vi "satellite simulator control.vi"() -> ()   [LabVIEW 2012]
uses:
  <vilib>/Utility/error.llb/DialogType.ctl
  <vilib>/DAQmx/create/channels.llb/DAQmx Create Channel (DO-Digital Output).vi
  <vilib>/vision/NI_Vision_Development_Module.lvlib
panel:
  in  "Pixel-Distance Ratio (pix/cm)":dbl=8.26
  in  "Remote Logger Status":bool
  in  "Downlink Object Data?":bool
  in  "Remote Port":u16=61557
  in  "Local Port":u16=61556
  in  "Remote Host":string="localhost"
  in  "broadcast":bool
  in  "Maintain Attitude":bool
  out "alpha":dbl
  out "Objects":T1(array[cluster]) {"Aspect Ratio" format="%.2f"; "Orientation" format="%.2f"; "Area" format="%.2f"; "Object Center"."Y" format="%.2f"; "Object Center"."X" format="%.2f"}
  in  "Y Center Correction":dbl
  in  "X Center Correction":dbl
  out "Offset Degree":dbl
  in  "Y Desired":dbl
  in  "X Desired":dbl
  out "Vx (cm/s)":dbl
  out "Vy (cm/s)":dbl
  in  "OK Button":bool
  out "Filtered Ohmega":dbl
  in  "Air Floating Status":bool
  in  "Control Freq":u32=20
  in  "Alpha Desired":dbl
  in  "STOP":bool caption="stop (F)"
  out "Image Out":T2(plugin-control)
  out "alpha (deg)":dbl
  out "dx (cm)":dbl
  out "dy (cm)":dbl
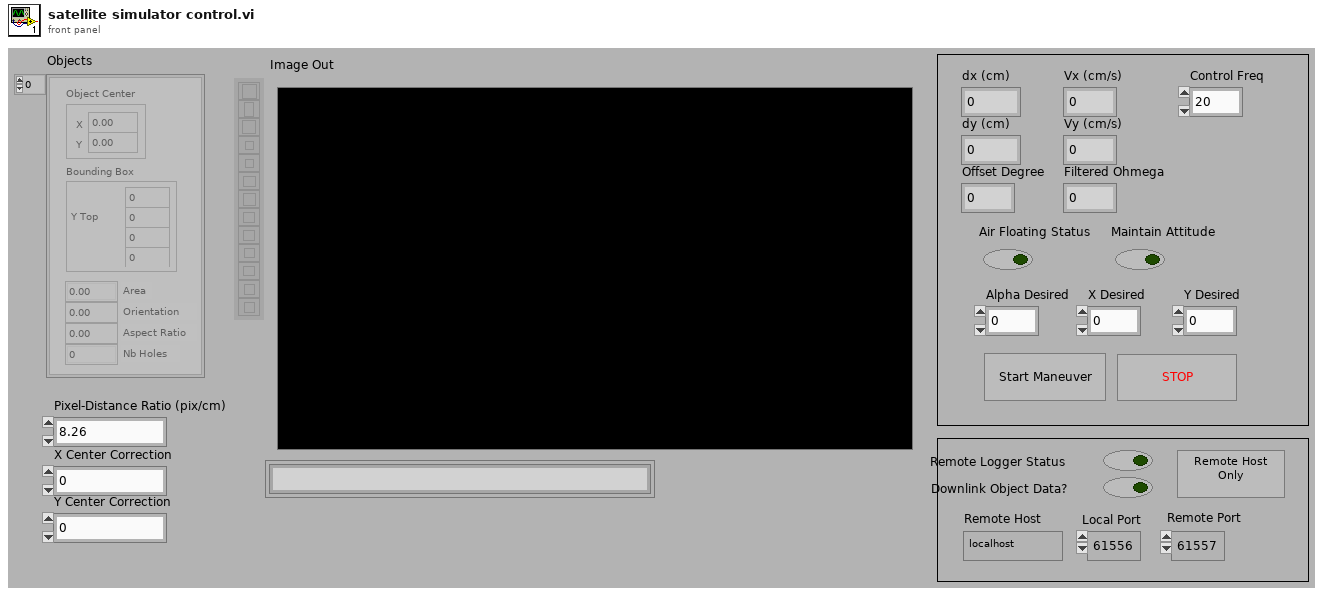
[diagram p1: front panel]
types:
  T1 = cluster{"Object Center":cluster{"X":sgl, "Y":sgl}, "Bounding Box":cluster{"X Left":i32, "Y Top":i32, "X Right":i32, "Y Bottom":i32}, "Area":sgl, "Orientation":sgl, "Aspect Ratio":sgl, "Nb Holes":i32}[]
  T2 = typedef "IMAQ Image.ctl" = refnum<image>
  T3 = typedef "DialogType.ctl" = u16
  T4 = cluster{"dx (cm)":dbl, "dy (cm)":dbl, "Offset Degree":dbl}
  T5 = cluster{"Objects":u16, "Threshold":i32, "Reject Border":bool, "Fill Holes":bool, "Min Object Size":bool, "Min Size":i32, "Max Object Size":bool, "Max Size":i32, "Show Search Area":bool, "Show Center":bool, "Show Bounding Box":bool}
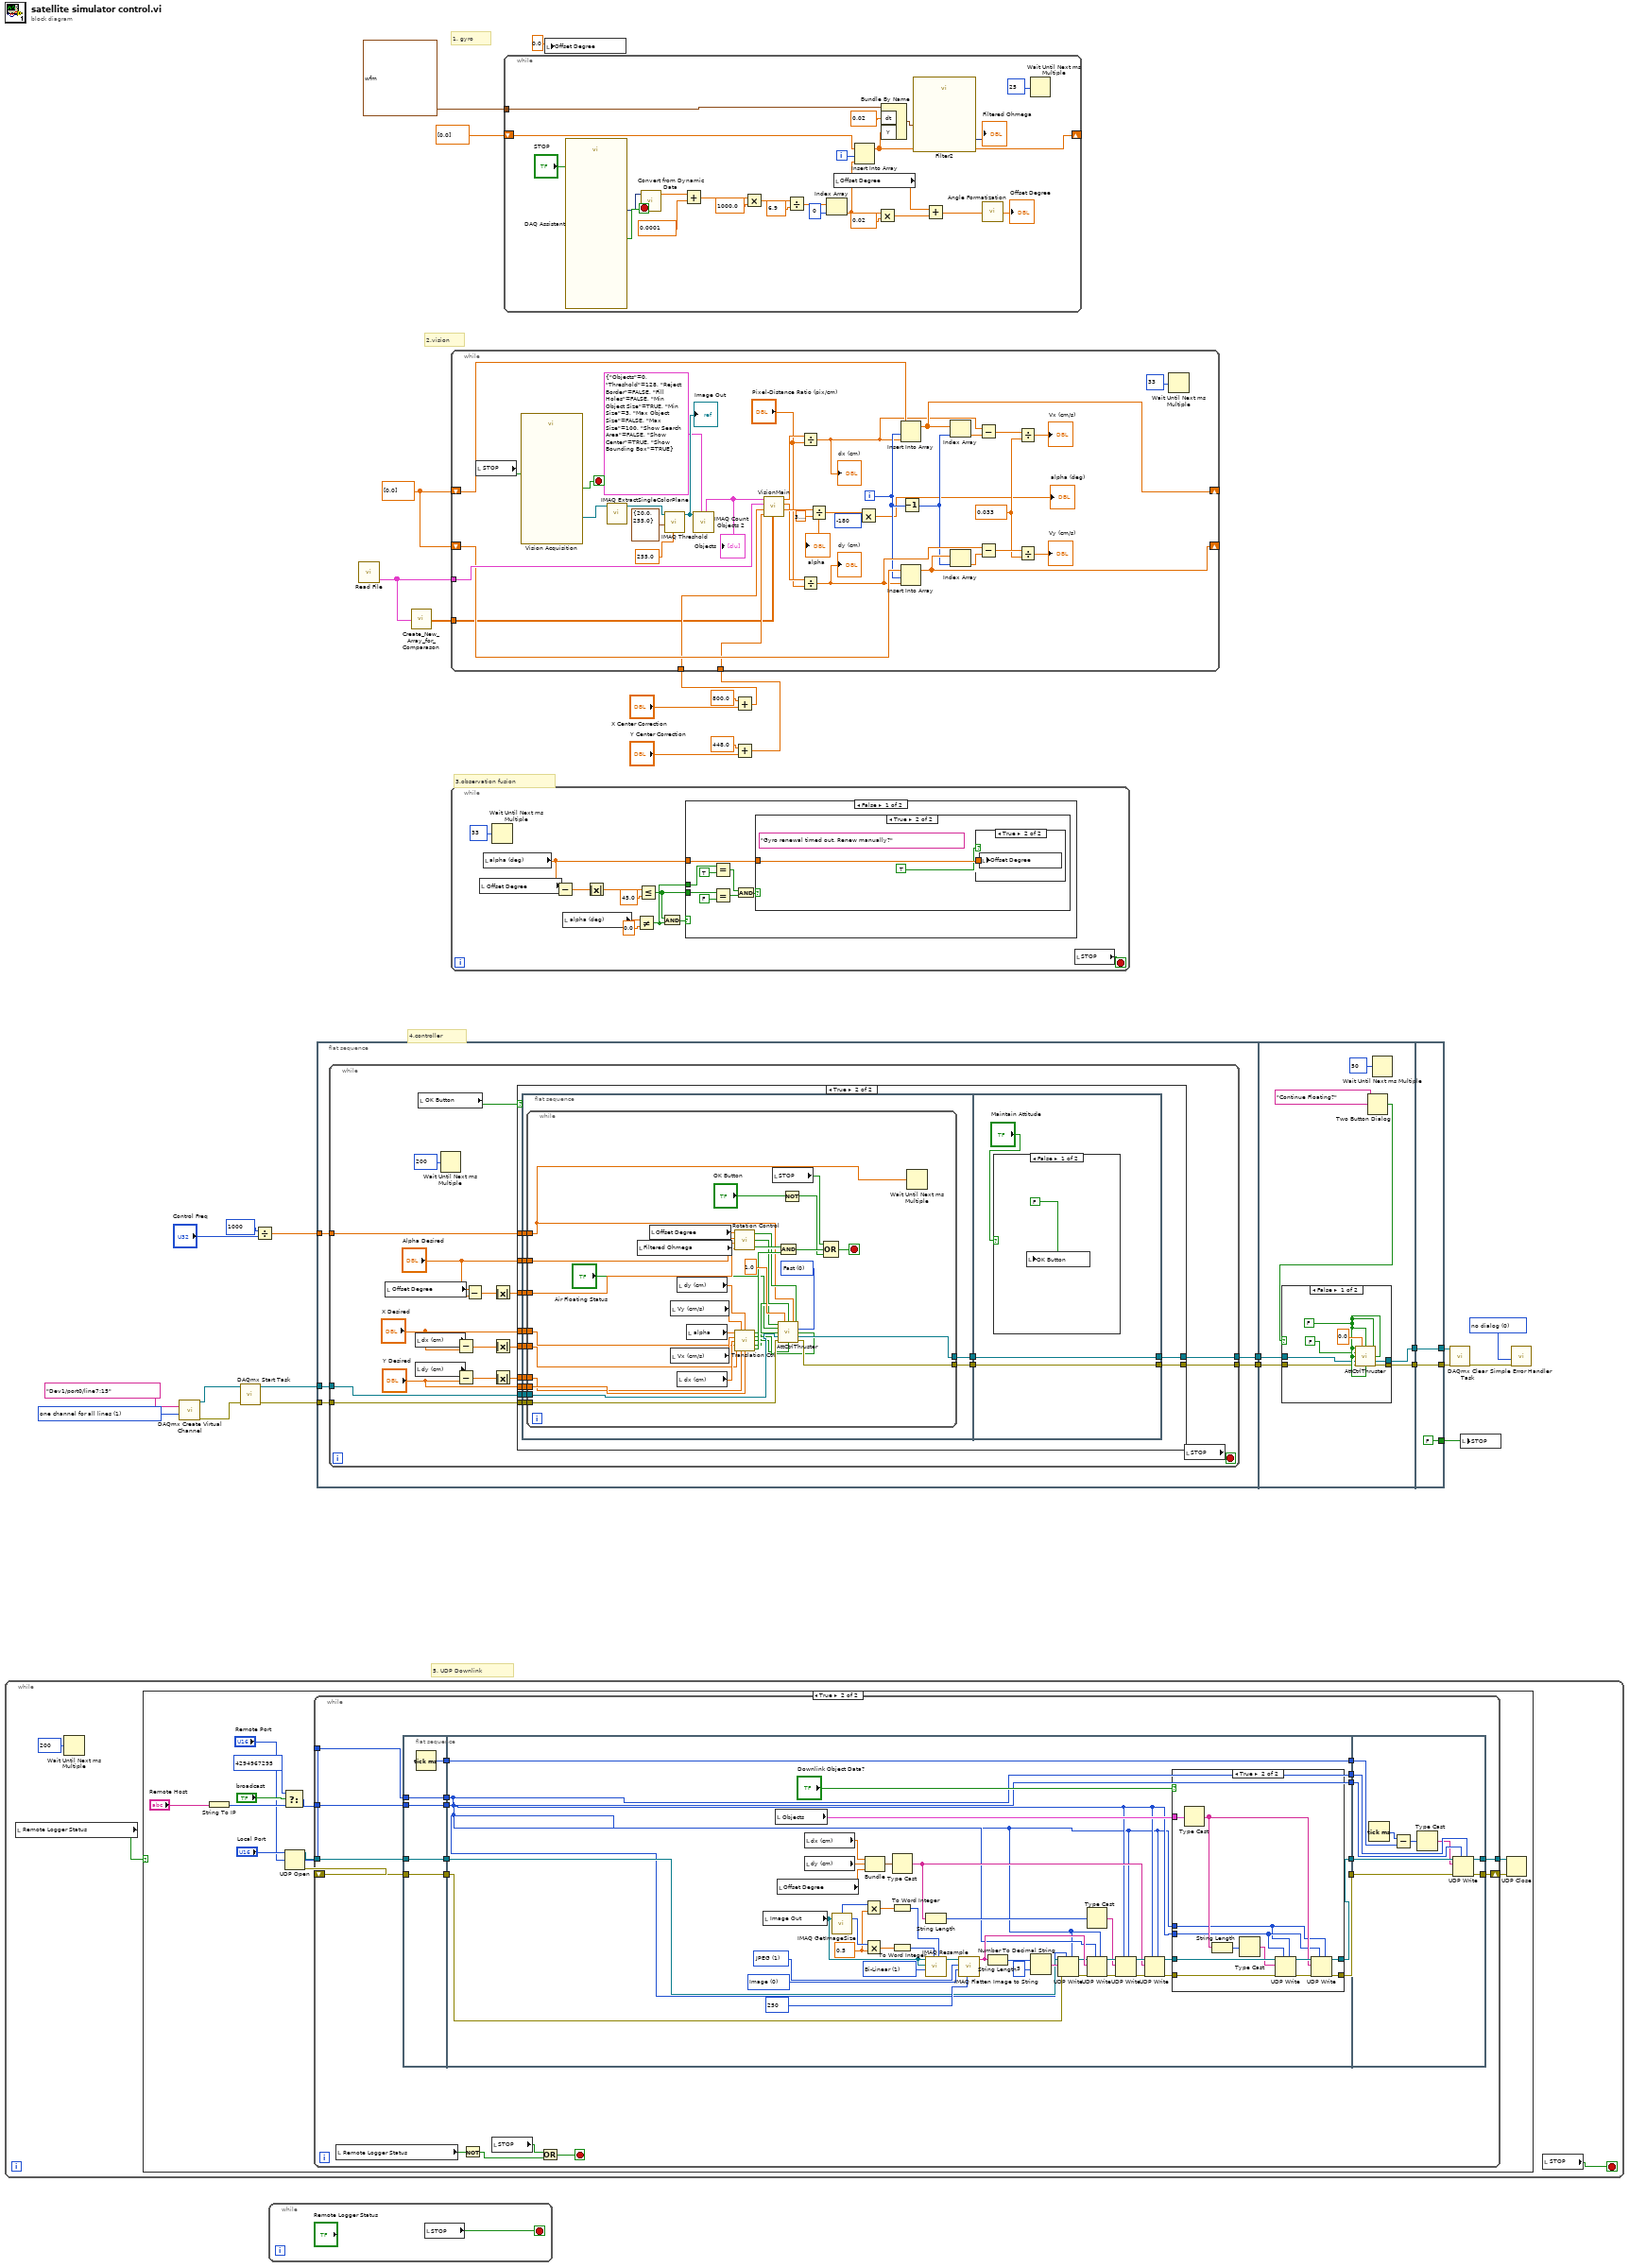
[diagram p0: block diagram]
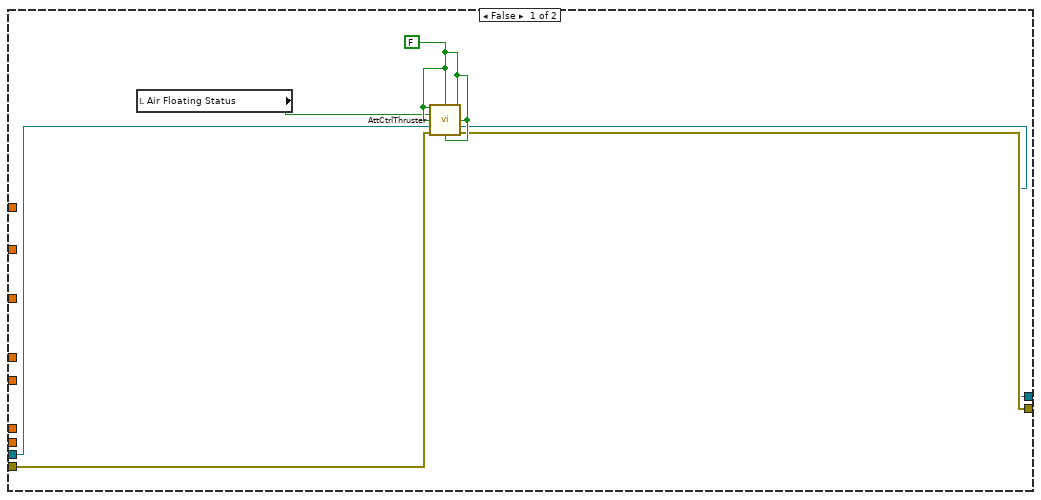
[diagram p4: hidden frame]
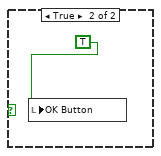
[diagram p5: hidden frame]
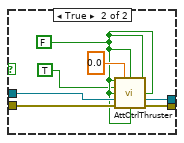
[diagram p6: hidden frame]
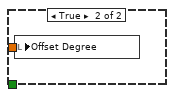
[diagram p9: hidden frame]
diagram:
  w25 = T3 0 items=["no dialog", "OK message", "continue or stop message", "OK message + warnings", "continue/stop + warnings"] ("type of dialog (OK msg:1)")
  w28 = 1 items=["one channel for each line", "one channel for all lines"] ("line grouping")
  w12 = dbl[] [0.0]
  # "5. UDP Downlink"
  # "4.controller"
  # "3.observation fusion"
  # "2.vision"
  # "1. gyro"
  n1 = while {
    stop <- w32 stop-if-true
    n2 = local read "Remote Logger Status"() -> (w33:bool)
    n3 = Wait Until Next ms Multiple(millisecond multiple=u32 200) -> ()  [unwired: 1 out]
    n4 = case shown="True" w33 {
      frame False {
      }
      frame True {
        n5 = String To IP(1:"Remote Host") -> (0:w41:u32)
        n6 = Select(t=u32 4294967295, s="broadcast", f=w41) -> (s? t:f=w38:u32)
        n7 = UDP Open(11:"Local Port") -> (port=w37:refnum<k16>, 0:w36:errorcluster)  [unwired: 1 in, 4 out]
        n8 = while {
          tunnel: "Remote Port" -> [w64]
          tunnel: w38 -> [w63]
          tunnel: w37 -> [w62]
          tunnel: [w60] -> w35
          shift-right: [w59] -> w34
          shift-left: w36 -> [w61]
          stop <- w48 stop-if-true
          n9 = local read "Remote Logger Status"() -> (w46:bool)
          n10 = flat-sequence {
            tunnel: w62 -> [w66]
            tunnel: w64 -> [w67]
            tunnel: w63 -> [w68]
            tunnel: w61 -> [w69]
            tunnel: [w69] -> w58
            tunnel: [w68] -> w57
            tunnel: [w67] -> w56
            tunnel: [w66] -> w55
            tunnel: [w65] -> w54
            tunnel: [w89] -> w53
            tunnel: [w88] -> w52
            tunnel: w58 -> [w107]
            tunnel: w57 -> [w71]
            tunnel: w56 -> [w70]
            tunnel: w55 -> [w91]
            tunnel: [w90] -> w51
            tunnel: w54 -> [w90]
            tunnel: [w70] -> w50
            tunnel: [w71] -> w49
            tunnel: [w131] -> w60
            tunnel: [w125] -> w59
            tunnel: w53 -> [w126]
            tunnel: w52 -> [w132]
            tunnel: w51 -> [w133]
            tunnel: w50 -> [w130]
            tunnel: w49 -> [w129]
            frame #0 {
              n11 = Tick Count (ms)() -> (millisecond timer value=w65:u32)
            }
            frame #1 {
              w95 = u32 1 items=["Zero Order", "Bi-Linear", "Quadratic", "Cubic Spline"] ("Interpolation Type")
              w96 = 0.5
              w104 = 0 items=["Image", "Image and Vision Info", "Reference to Image"] ("Type of Flatten (Image and Vision Info)")
              w109 = 1 items=["None", "JPEG", "PACKED BINARY"] ("Compression (None)")
              n12 = local read "Image Out"() -> (w85:T2)
              n13 = local read "Objects"() -> (w86:T1)
              n14 = local read "Offset Degree"() -> (w82:dbl)
              n15 = local read "dx (cm)"() -> (w84:dbl)
              n16 = local read "dy (cm)"() -> (w83:dbl)
              n17 = call "IMAQ GetImageSize"("Image"=w85) -> ("Y Resolution"=w97:i32, "X Resolution"=w98:i32)  [unwired: 3 in, 1 out]
              n18 = Multiply(x=w98, y=w96) -> (x*y=w100:dbl)
              n19 = Multiply(x=w97, y=w96) -> (x*y=w102:dbl)
              n20 = Bundle("dx (cm)"=w84, "dy (cm)"=w83, "Offset Degree"=w82) -> (w81:T4)  [unwired: 1 in]
              n21 = To Word Integer(number=w100) -> (16bit integer=w99:i16)
              n22 = To Word Integer(number=w102) -> (16bit integer=w101:i16)
              n23 = Type Cast(x=w81) -> (*(type *) &x=w72:string)  [unwired: 1 in]
              n24 = String Length(string=w72) -> (length=w74:i32)
              n25 = call "IMAQ Resample"("X Resolution"=w99, "Y Resolution"=w101, "Interpolation Type"=w95, "Image Dst"=w85, "Image Src"=w85) -> ("Image Dst Out"=w103:T2)  [unwired: 5 in, 1 out]
              n26 = call "IMAQ Flatten Image to String"("Quality (750)"=250, "Type of Flatten (Image and Vision Info)"=w104, "Compression (None)"=w109, "Image"=w103) -> ("Data String"=w108:string)  [unwired: 6 in, 1 out]
              n27 = String Length(string=w108) -> (length=w94:i32)
              n28 = Number To Decimal String(number=w94, width (-)=i16 5) -> (decimal integer string=w93:string)
              n29 = UDP Write(address=w71, port or service name=w70, connection ID=w91, data in=w93, 8:w107) -> (error out=w106:errorcluster, 3:w105:refnum<k16>)  [unwired: 1 out]
              n30 = Type Cast(x=w74) -> (*(type *) &x=w73:string)  [unwired: 1 in]
              n31 = UDP Write(address=w71, port or service name=w70, connection ID=w105, data in=w108, 8:w106) -> (error out=w79:errorcluster, 3:w80:refnum<k16>)  [unwired: 1 out]
              n32 = UDP Write(address=w71, port or service name=w70, connection ID=w80, data in=w73, 8:w79) -> (error out=w78:errorcluster, 3:w76:refnum<k16>)  [unwired: 1 out]
              n33 = UDP Write(address=w71, port or service name=w70, connection ID=w76, data in=w72, 8:w78) -> (error out=w77:errorcluster, 3:w75:refnum<k16>)  [unwired: 1 out]
              n34 = case shown="True" "Downlink Object Data?" {
                tunnel: w86 -> [_ w124]
                tunnel: w77 -> [w112 w122]
                tunnel: [w112 w120] -> w89
                tunnel: w75 -> [w111 w119]
                tunnel: [w111 w117] -> w88
                tunnel: w71 -> [_ w114]
                tunnel: w70 -> [_ w113]
                frame False {
                }
                frame True {
                  n35 = Type Cast(x=w124) -> (*(type *) &x=w115:string)  [unwired: 1 in]
                  n36 = String Length(string=w115) -> (length=w123:i32)
                  n37 = Type Cast(x=w123) -> (*(type *) &x=w116:string)  [unwired: 1 in]
                  n38 = UDP Write(address=w114, port or service name=w113, connection ID=w119, data in=w116, 8:w122) -> (error out=w121:errorcluster, 3:w118:refnum<k16>)  [unwired: 1 out]
                  n39 = UDP Write(address=w114, port or service name=w113, connection ID=w118, data in=w115, 8:w121) -> (error out=w120:errorcluster, 3:w117:refnum<k16>)  [unwired: 1 out]
                }
              }
            }
            frame #2 {
              n40 = Tick Count (ms)() -> (millisecond timer value=w134:u32)
              n41 = Subtract(x=w134, y=w133) -> (x-y=w128:u32)
              n42 = Type Cast(x=w128) -> (*(type *) &x=w127:string)  [unwired: 1 in]
              n43 = UDP Write(address=w129, port or service name=w130, connection ID=w132, data in=w127, 8:w126) -> (error out=w125:errorcluster, 3:w131:refnum<k16>)  [unwired: 1 out]
            }
          }
          n44 = Not(x=w46) -> (.not. x?=w45:bool)
          n45 = local read "STOP"() -> (w47:bool)
          n46 = Or(x=w47, y=w45) -> (x .or. y?=w48:bool)
        }
        n47 = UDP Close(connection ID=w35, 8:w34) -> ()  [unwired: 2 out]
      }
    }
    n48 = local read "STOP"() -> (w32:bool)
  }
  n49 = call-poly <vilib>:"DAQmx Create Virtual Channel.vi"("lines"=tag "Dev1/port0/line7:15" ("Lines"), "line grouping"=w28) -> ("task out"=w26:refnum<k21>, "error out"=w27:errorcluster)  [unwired: 12 in]
  n50 = call <vilib>:"DAQmx Start Task.vi"("task/channels in"=w26, "error in"=w27) -> ("task out"=w21:refnum<k21>, "error out"=w20:errorcluster)  [unwired: 12 in]
  n51 = Divide(x=u32 1000 ("milliseconds to wait"), y="Control Freq") -> (x/y=w17:dbl)
  n52 = while {
    stop <- w135 stop-if-true
    n53 = local read "STOP"() -> (w135:bool)
  }
  n54 = flat-sequence {
    tunnel: w21 -> [w140]
    tunnel: w20 -> [w139]
    tunnel: w17 -> [w136]
    tunnel: [w138] -> w16
    tunnel: [w137] -> w15
    tunnel: w16 -> [w236]
    tunnel: w15 -> [w234]
    tunnel: [w235] -> w5
    tunnel: [w233] -> w4
    tunnel: [w252] -> w18
    tunnel: [w253] -> w19
    tunnel: w5 -> [w253]
    tunnel: w4 -> [w252]
    tunnel: [FALSE] -> w3
    frame #0 {
      n55 = while {
        tunnel: w140 -> [w160]
        tunnel: w139 -> [w159]
        tunnel: [w158] -> w138
        tunnel: [w157] -> w137
        tunnel: w136 -> [w142]
        stop <- w156 stop-if-true
        n56 = local read "Offset Degree"() -> (w155:dbl)
        n57 = local read "dx (cm)"() -> (w151:dbl)
        n58 = local read "dy (cm)"() -> (w147:dbl)
        n59 = local read "OK Button"() -> (w143:bool)
        n60 = Wait Until Next ms Multiple(millisecond multiple=u32 200) -> ()  [unwired: 1 out]
        n61 = Subtract(x=w151, y="X Desired") -> (x-y=w149:dbl)
        n62 = Subtract(x=w147, y="Y Desired") -> (x-y=w145:dbl)
        n63 = Subtract(x=w155, y="Alpha Desired") -> (x-y=w153:dbl)
        n64 = Absolute Value(x=w153) -> (abs(x)=w152:dbl)
        n65 = Absolute Value(x=w149) -> (abs(x)=w148:dbl)
        n66 = Absolute Value(x=w145) -> (abs(x)=w144:dbl)
        n67 = case shown="True" w143 {
          tunnel: w160 -> [w164 w179]
          tunnel: w159 -> [w163 w178]
          tunnel: [w162 w177] -> w158
          tunnel: [w161 w176] -> w157
          tunnel: w142 -> [_ w175]
          tunnel: "Alpha Desired" -> [_ w174]
          tunnel: w152 -> [_ w173]
          tunnel: "X Desired" -> [_ w172]
          tunnel: w148 -> [_ w171]
          tunnel: "Y Desired" -> [_ w170]
          tunnel: w144 -> [_ w169]
          frame False {
            w166 = FALSE
            n68 = local read "Air Floating Status"() -> (w165:bool)
            n69 = call "AttCtrlThruster.vi"("ctclk"=w166, "Up"=w166, "clkwis"=w166, "Float"=w165, "Left"=w166, "Right"=w166, "task in"=w164, "error in"=w163, "Down"=w166) -> ("task out"=w161:refnum<k21>, "error out"=w162:errorcluster)  [unwired: 5 in]
          }
          frame True {
            n70 = flat-sequence {
              tunnel: w179 -> [w190]
              tunnel: w178 -> [w189]
              tunnel: w175 -> [w186]
              tunnel: w174 -> [w185]
              tunnel: w173 -> [w184]
              tunnel: w172 -> [w183]
              tunnel: w171 -> [w182]
              tunnel: w170 -> [w181]
              tunnel: w169 -> [w180]
              tunnel: [w188] -> w168
              tunnel: [w187] -> w167
              tunnel: [w226] -> w176
              tunnel: [w227] -> w177
              tunnel: w168 -> [w227]
              tunnel: w167 -> [w226]
              frame #0 {
                n71 = while {
                  tunnel: w190 -> [w224]
                  tunnel: w189 -> [w223]
                  tunnel: [w221] -> w188
                  tunnel: [w222] -> w187
                  tunnel: w186 -> [w192]
                  tunnel: w185 -> [w202]
                  tunnel: w184 -> [w217]
                  tunnel: w183 -> [w201]
                  tunnel: w182 -> [w212]
                  tunnel: w181 -> [w200]
                  tunnel: w180 -> [w199]
                  stop <- w218 stop-if-true
                  w208 = u16 0 items=["Fast", "Slow"] ("Angular Acceleration")
                  n72 = local read "Filtered Ohmega"() -> (w216:dbl)
                  n73 = local read "Offset Degree"() -> (w215:dbl)
                  n74 = local read "Vy (cm/s)"() -> (w211:dbl)
                  n75 = local read "Vx (cm/s)"() -> (w214:dbl)
                  n76 = local read "dy (cm)"() -> (w210:dbl)
                  n77 = local read "dx (cm)"() -> (w213:dbl)
                  n78 = local read "alpha"() -> (w196:dbl)
                  n79 = call "Rotation Control.vi"("Filtered Ohmega"=w216, "Original Difference"=w217, "Alpha Desired"=w202, "Alpha In"=w215) -> ("Maneuver Complete?"=w195:bool, "Counter-ClkWise Rot Ctrl"=w194:bool, "Clockwise Rot Ctrl"=w193:bool)
                  n80 = call "Translation Ctrl.vi"("Alpha"=w196, "Filtered Speed Y"=w211, "Y In"=w210, "Filtered Speed X"=w214, "X In"=w213, "X Desired"=w201, "Original Difference X"=w212, "Original Difference Y"=w199, "Y Desired"=w200) -> ("Left"=w206:bool, "Right"=w205:bool, "Down"=w204:bool, "Up"=w203:bool, "Maneuver Complete?"=w207:bool)  [unwired: 2 in]
                  n81 = local read "STOP"() -> (w219:bool)
                  n82 = call "AttCtrlThruster.vi"("ctclk"=w194, "Duty Cycle"=1.0, "Up"=w203, "Period"=w192, "clkwis"=w193, "Float"="Air Floating Status", "Angular Acceleration"=w208, "Left"=w206, "Right"=w205, "task in"=w224, "error in"=w223, "Down"=w204) -> ("task out"=w222:refnum<k21>, "error out"=w221:errorcluster)  [unwired: 2 in]
                  n83 = And(x=w195, y=w207) -> (x .and. y?=w209:bool)
                  n84 = Not(x="OK Button") -> (.not. x?=w197:bool)
                  n85 = Compound Arithmetic op=OR(w219, w209, w197) -> (w218:bool)
                  n86 = Wait Until Next ms Multiple(millisecond multiple=w192) -> ()  [unwired: 1 out]
                }
              }
              frame #1 {
                n87 = case shown="False" "Maintain Attitude" {
                  frame False {
                    n88 = local write "OK Button"(FALSE) -> ()
                  }
                  frame True {
                    n89 = local write "OK Button"(TRUE) -> ()
                  }
                }
              }
            }
          }
        }
        n90 = local read "STOP"() -> (w156:bool)
      }
    }
    frame #1 {
      n91 = Two Button Dialog(message="Continue Floating?") -> (T button?=w230:bool)  [unwired: 2 in]
      n92 = case shown="False" w230 {
        tunnel: w236 -> [w239 w250]
        tunnel: [w237 w249] -> w235
        tunnel: w234 -> [w240 w248]
        tunnel: [w238 w247] -> w233
        frame False {
          w242 = FALSE
          n93 = call "AttCtrlThruster.vi"("ctclk"=w242, "Duty Cycle"=0.0, "Up"=w242, "clkwis"=w242, "Float"=FALSE, "Left"=w242, "Right"=w242, "task in"=w240, "error in"=w239, "Down"=w242) -> ("task out"=w238:refnum<k21>, "error out"=w237:errorcluster)  [unwired: 4 in]
        }
        frame True {
          w245 = FALSE
          n94 = call "AttCtrlThruster.vi"("ctclk"=w245, "Duty Cycle"=0.0, "Up"=w245, "clkwis"=w245, "Float"=TRUE, "Left"=w245, "Right"=w245, "task in"=w248, "error in"=w250, "Down"=w245) -> ("task out"=w247:refnum<k21>, "error out"=w249:errorcluster)  [unwired: 4 in]
        }
      }
      n95 = Wait Until Next ms Multiple(millisecond multiple=u32 50) -> ()  [unwired: 1 out]
    }
    frame #2 {
    }
  }
  n96 = call "Read File.vi"() -> ("Objects"=w1:T1)  [unwired: 1 in, 1 out]
  n97 = call "Create_New_Array_for_Comparason.vi"("Captured Plots"=w1) -> ("Generated Distance Array"=w2:dbl[][])
  n98 = while {
    stop <- w264 stop-if-true
    n99 = local read "Offset Degree"() -> (w263:dbl)
    n100 = local read "alpha (deg)"() -> (w259:dbl)
    n101 = Wait Until Next ms Multiple(millisecond multiple=u32 33) -> ()  [unwired: 1 out]
    n102 = Subtract(x=w263, y=w259) -> (x-y=w262:dbl)
    n103 = local read "alpha (deg)"() -> (w257:dbl)
    n104 = Absolute Value(x=w262) -> (abs(x)=w261:dbl)
    n105 = Not Equal?(x=w257, y=0.0) -> (x != y?=w255:bool)
    n106 = Less Or Equal?(x=w261, y=45.0) -> (x <= y?=w254:bool)
    n107 = And(x=w254, y=w255) -> (x .and. y?=w258:bool)
    n108 = case shown="False" w258 {
      tunnel: w259 -> [w266 w277]
      tunnel: w255 -> [w268 _]
      tunnel: w254 -> [w267 _]
      frame False {
        n109 = Equal?(x=w268, y=TRUE) -> (x = y?=w272:bool)
        n110 = Equal?(x=w267, y=FALSE) -> (x = y?=w271:bool)
        n111 = And(x=w272, y=w271) -> (x .and. y?=w269:bool)
        n112 = case shown="True" w269 {
          tunnel: w266 -> [_ w275]
          frame False {
          }
          frame True {
            (unwired) "Gyro renewal timed out. Renew manually?" ("message")
            n113 = case shown="True" TRUE {
              tunnel: w275 -> [_ w276]
              frame False {
              }
              frame True {
                n114 = local write "Offset Degree"(w276) -> ()
              }
            }
          }
        }
      }
      frame True {
        n115 = local write "Offset Degree"(w277) -> ()
      }
    }
    n116 = local read "STOP"() -> (w264:bool)
  }
  n117 = while {
    shift-right: [w285] -> _
    shift-left: dbl[] [0.0] -> [w286]
    tunnel: waveform(dbl) {"t0"=timestamp(0 s since 1904-01-01), "dt"=1.0, "Y"=[]} ("waveform") -> [w283]
    i -> [w284]
    stop <- w301 stop-if-true
    n118 = call "DAQ Assistant"("stop (F)"="STOP") -> ("data"=w293:dynamicdata, "stopped"=w301:bool)  [unwired: 15 in, 2 out]
    n119 = call "Convert from Dynamic Data"("Dynamic Data Type"=w293) -> ("Array"=w291:dbl[])  [unwired: 3 in]
    n120 = Add(x=w291, y=0.0001) -> (x+y=w289:dbl[])
    n121 = Multiply(x=w289, y=1000.0) -> (x*y=w300:dbl[])
    n122 = Divide(x=w300, y=6.9) -> (x/y=w294:dbl[])
    n123 = Index Array(array=w294, index=0) -> (element=w279:dbl)
    n124 = local read "Offset Degree"() -> (w288:dbl)
    n125 = Insert Into Array(array=w286, index=w284, new element=w279) -> (w285:dbl[])
    n126 = Multiply(x=w279, y=0.02) -> (x*y=w295:dbl)
    n127 = Bundle By Name(cluster=w283, "dt"=0.02, "Y"=w285) -> (w282:waveform(dbl))
    n128 = call "Filter2"("Signal"=w282) -> ("Filtered Signal"=→"Filtered Ohmega":dynamicdata)  [unwired: 9 in, 1 out]
    n129 = Add(x=w288, y=w295) -> (x+y=w281:dbl)
    n130 = call "Angle Formatization.vi"("Alpha"=w281) -> ("Alpha Formatized"=→"Offset Degree":dbl)
    n131 = Wait Until Next ms Multiple(millisecond multiple=u32 25 ("y")) -> ()  [unwired: 1 out]
  }
  n132 = local write "Offset Degree"(0.0 ("y")) -> ()
  n133 = Add(x=800.0 ("c_x"), y="X Center Correction") -> (x+y=w9:dbl)
  n134 = Add(x=448.0 ("c_y"), y="Y Center Correction") -> (x+y=w6:dbl)
  n135 = while {
    tunnel: w1 -> [w328]
    shift-right: [w325] -> _
    shift-left: w12 -> [w326]
    shift-right: [w314] -> _
    shift-left: w12 -> [w317]
    tunnel: w6 -> [w307]
    tunnel: w9 -> [w306]
    tunnel: w2 -> [w303]
    i -> [w316]
    stop <- w339 stop-if-true
    w310 = 0.033 ("y")
    n136 = local read "STOP"() -> (w330:bool)
    n137 = call "Vision Acquisition"("Stop (F)"=w330) -> ("Image Out"=w334:T2, "Stopped"=w339:bool)  [unwired: 24 in, 1 out]
    n138 = call "IMAQ ExtractSingleColorPlane"("Image Src"=w334) -> ("Image Dst Out"=w338:T2)  [unwired: 9 in, 1 out]
    n139 = call "IMAQ Threshold"("Replace Value"=sgl 255.0 ("replace value"), "Range"=cluster{"lower value":sgl, "upper value":sgl} {"lower value"=20.0, "upper value"=255.0} ("threshold"), "Image Src"=w338) -> ("Image Dst Out"=w335:T2)  [unwired: 7 in, 1 out]
    "Image Out" <- w335
    n140 = call "IMAQ Count Objects 2"("Settings"=T5 {"Objects"=0, "Threshold"=128, "Reject Border"=FALSE, "Fill Holes"=FALSE, "Min Object Size"=TRUE, "Min Size"=3, "Max Object Size"=FALSE, "Max Size"=100, "Show Search Area"=FALSE, "Show Center"=TRUE, "Show Bounding Box"=TRUE}, "Image"=w335) -> ("Objects"=w329:T1)  [unwired: 5 in, 4 out]
    "Objects" <- w329
    n141 = call "VisionMain.vi"("Generated Distance Array"=w303, "Y Center"=w307, "X Center"=w306, "Original Plots"=w328, "Plots Captured"=w329) -> ("alpha"=w327:dbl, "dy"=w323:dbl, "dx"=w318:dbl)  [unwired: 4 in]
    "alpha" <- w327
    n142 = Divide(x=w318, y="Pixel-Distance Ratio (pix/cm)") -> (x/y=w313:dbl)
    "dx (cm)" <- w313
    n143 = Divide(x=w323, y="Pixel-Distance Ratio (pix/cm)") -> (x/y=w322:dbl)
    "dy (cm)" <- w322
    n144 = Divide(x=w327, y=3.141592653589793) -> (x/y=w332:dbl)
    n145 = Multiply(x=w332, y=-180) -> (x*y=→"alpha (deg)":dbl)
    n146 = Insert Into Array(array=w317, index=w316, new element=w313) -> (w314:dbl[])
    n147 = Insert Into Array(array=w326, index=w316, new element=w322) -> (w325:dbl[])
    n148 = Decrement(x=w316) -> (x-1=w315:i32)
    n149 = Index Array(array=w314, index=w315) -> (element=w312:dbl)
    n150 = Index Array(array=w325, index=w315) -> (element=w324:dbl)
    n151 = Subtract(x=w313, y=w312) -> (x-y=w311:dbl)
    n152 = Subtract(x=w322, y=w324) -> (x-y=w321:dbl)
    n153 = Divide(x=w311, y=w310) -> (x/y=→"Vx (cm/s)":dbl)
    n154 = Divide(x=w321, y=w310) -> (x/y=→"Vy (cm/s)":dbl)
    n155 = Wait Until Next ms Multiple(millisecond multiple=u32 33) -> ()  [unwired: 1 out]
  }
  n156 = call <vilib>:"DAQmx Clear Task.vi"("task in"=w18, "error in"=w19) -> ("error out"=w24:errorcluster)  [unwired: 13 in]
  n157 = local write "STOP"(w3) -> ()
  n158 = call <vilib>:"Simple Error Handler.vi"("type of dialog (OK msg:1)"=w25, "error in (no error)"=w24) -> ()  [unwired: 3 in, 5 out]
